vi "PLC_PROXY_MAIN.vi"() -> ()   [LabVIEW 2020]
uses:
  PLC_PROXY/FGV/connection_references/FGV_PROXY_connection_references.ctl
  PLC_PROXY/STATION/station.ctl
  PLC_PROXY/ini/typedef/PROXY_all_config_info.ctl
  PLC_PROXY/ini/typedef/PROXY_main_ini_file.ctl
  PLC_PROXY/queues/typedef/PROXY_queue_refnums.ctl
  PLC_PROXY/queues/typedef/STATION_queue_element.ctl
  PLC_PROXY/STATION/ST_SQL_sequence_state.ctl
  PLC_PROXY/FGV/error_buffer/FGV_PROXY_error_buffer.ctl
  PLC_PROXY/MAIN/PROXY_event_structure_shift_register.ctl
  PLC_PROXY/FGV/DIAGNOSTICS_records_display/FGV_PROXY_DIAGNOSTICS_records_display.ctl
  PLC_PROXY/FGV/DIAGNOSTICS_connection_indicators/FGV_PROXY_connection_indicators.ctl
  PLC_PROXY/FGV/DIAGNOSTICS_message_history_buffer/FGV_PROXY_DIAGNOSTICS_message_history_buffer.ctl
  PLC_PROXY/FGV/SQL_part_ID_buffer/FGV_SQL_part_ID_buffer.ctl
  PLC_PROXY/FGV/SQL_pinion_ID_buffer/FGV_SQL_pinion_ID_buffer.ctl
  PLC_PROXY/FGV/SQL_batch_ID_buffer/FGV_SQL_batch_ID_buffer.ctl
  PLC_PROXY/MAIN/reference_change_listener/PROXY_REF_CHG_sequence_state.ctl
  _misc/NotifyIcon/TypeDefs/NotifyIcon Event Registration Actions.ctl
  _misc/NotifyIcon/TypeDefs/NotifyIcon Events.ctl
  PLC_PROXY/FGV/reference_change_connection/FGV_PROXY_REF_CHG_connection.ctl
  System.Windows.Forms
  _misc/AULocalize/SubVIs/Get Localized Phrase Compact Interface 2D.vi
  _misc/AULocalize/SubVIs/RegisterVI.vi
  _misc/AULocalize/SubVIs/Get Localized Phrase Compact Interface 0D.vi
panel:
  out "app_title":string caption="A603 - PLC Proxy"
  out "SQL_connections_indicator_global":bool=TRUE caption="SQL Connections Status:"
  out "PLC_connections_indicator_global":bool=TRUE caption="PLC Connections Status:"
  in  "STOP":bool
  out "error_indicator_global":bool caption="Application Status:"
  in  "main_tab":enum32{"Diagnostics", "Errors"}(tab)
  in  "DIAGNOSTICS_save_log":bool
  in  "DIAGNOSTICS_all_stations_messages":bool
  in  "DIAGNOSTICS_records":i32(listbox)
  in  "main_error":i32(listbox)
  in  "ERRORS_clear":bool
  out "error_indicator_tab":bool
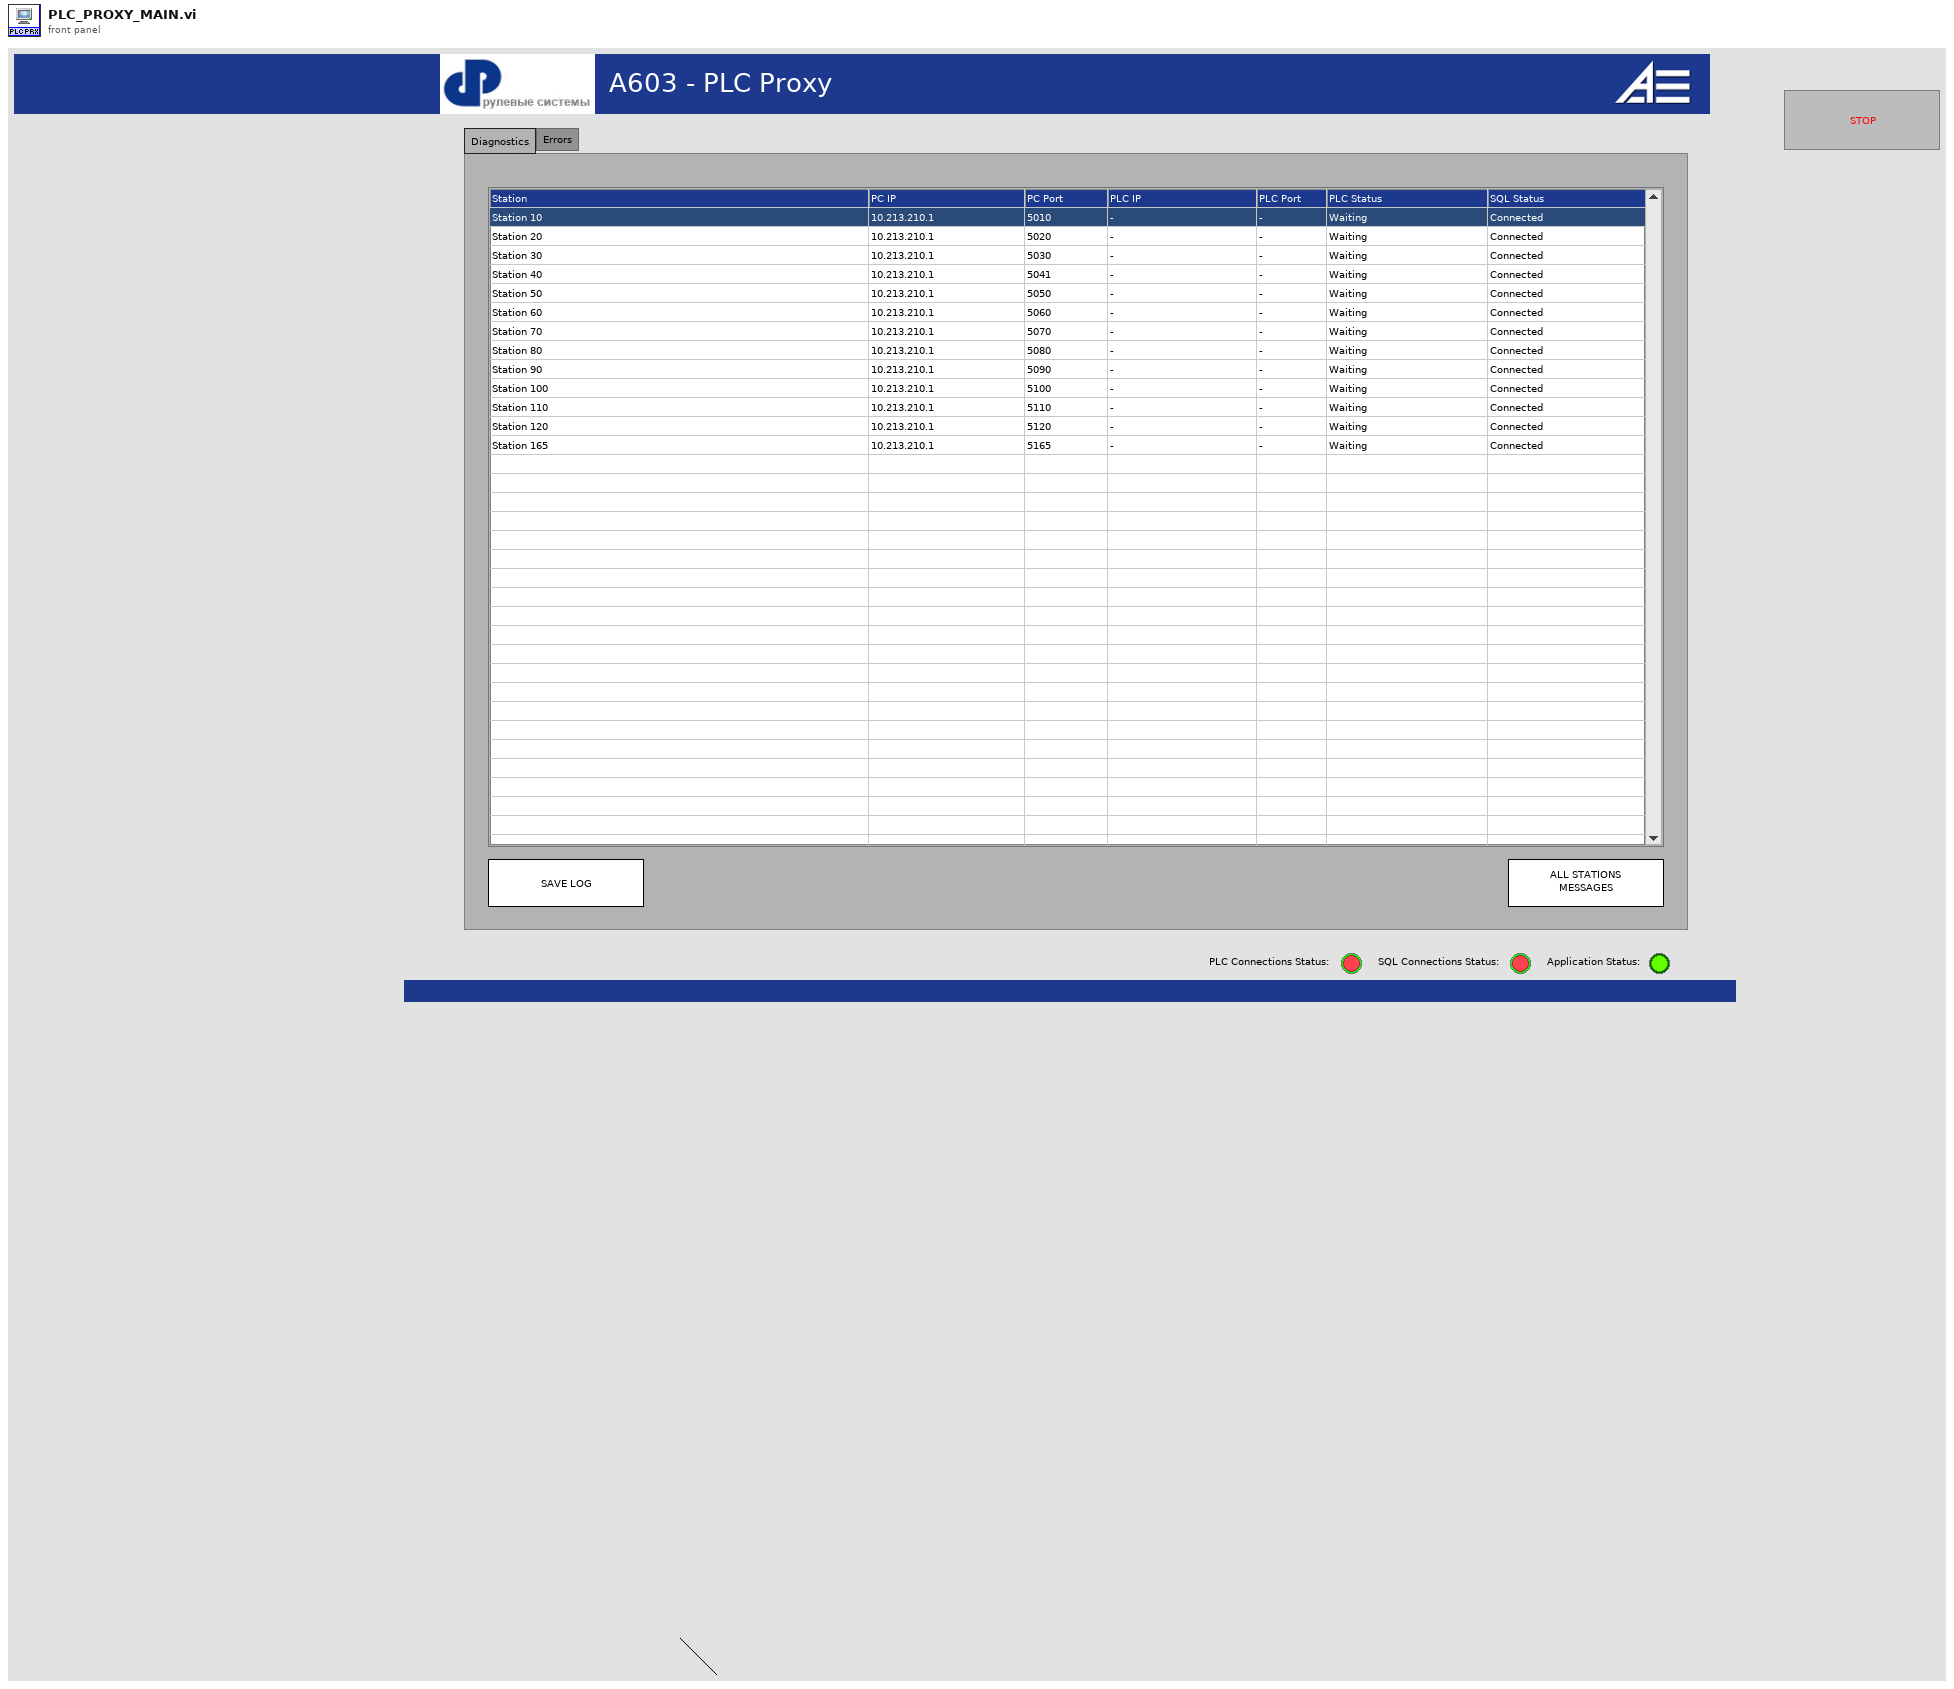
[diagram p1: front panel]
types:
  T1 = typedef "NotifyIcon Events.ctl" = enum16{"BalloonTipClicked", "BalloonTipClosed", "BalloonTipShown", "Click", "Disposed", "DoubleClick", "MouseClick", "MouseDoubleClick", "MouseDown", "MouseMove", "MouseUp", "MenuItemClick", "MenuItemSelect"}
  T2 = typedef "NotifyIcon Event Registration Actions.ctl" = enum16{"Initial Event Registration", "Add to Event Registration", "Destroy Events and Re-register"}
  T3 = typedef "PROXY_REF_CHG_sequence_state.ctl" = enum16{"initialize", "wait_for_connection", "handle_message", "error", "stop"}
  T4 = typedef "FGV_SQL_batch_ID_buffer.ctl" = enum16{"initialize", "get_ID_for_number"}
  T5 = typedef "station.ctl" = enum16{"STATION_10", "STATION_20", "STATION_30", "STATION_40", "STATION_50", "STATION_60", "STATION_70", "STATION_80", "STATION_90", "STATION_100", "STATION_110", "STATION_120", "STATION_165", "MAIN"}
  T6 = typedef "FGV_SQL_pinion_ID_buffer.ctl" = enum16{"initialize", "buffer_pinion_ID", "buffer_pinion_ID_SQL", "get_ID_for_name"}
  T7 = typedef "FGV_SQL_part_ID_buffer.ctl" = enum16{"initialize", "buffer_serial_ID", "get_ID_for_name"}
  T8 = typedef "FGV_PROXY_DIAGNOSTICS_message_history_buffer.ctl" = enum16{"initialize", "add_TCP_PLC_to_PC", "add_TCP_PC_to_PLC", "add_SQL_PC_to_DB", "add_SQL_transaction", "add_SQL_DB_to_PC", "get_station", "get_all", "clear_station", "clear_all", "save_log"}
  T9 = typedef "FGV_PROXY_connection_indicators.ctl" = enum16{"initialize", "SQL_conn_ind_update", "PLC_conn_ind_update"}
  T10 = typedef "FGV_PROXY_DIAGNOSTICS_records_display.ctl" = enum16{"initialize", "set_PLC_IP", "set_PLC_Port", "set_PLC_connection_status", "set_SQL_connection_status", "get_all_info"}
  T11 = typedef "PROXY_event_structure_shift_register.ctl" = cluster{"REF_EDIT_clicked_row":i32, "REF_EDIT_selected_row":i32, "SQL_EDIT_clicked_row":i32, "SQL_EDIT_selected_row":i32, "ARCH_EDIT_selected_row":i32, "ARCH_EDIT_clicked_row":i32, "USER_EDIT_selected_row":i32, "USER_EDIT_clicked_row":i32, "REPORT_GEAR_toggle_all_results":bool}
  T12 = typedef "FGV_PROXY_error_buffer.ctl" = enum16{"initialize", "clear", "display", "get_status"}
  T13 = typedef "PROXY_all_config_info.ctl" = cluster{"main_ini_file":T14, "SQL Password":string, "queue_refnums":T15, "number_of_stations":i32}
  T14 = typedef "PROXY_main_ini_file.ctl" = cluster{"SQL Driver":string, "SQL Server":string, "SQL Database":string, "SQL UID":string, "Reference table":string, "Reference history":string, "Archivisation CFG table":string, "Archivisation CFG history":string, "Archivisation Audit table":string, "User table":string, "User history":string, "default language":string, "REF CHG listener IP":string, "REF CHG listener port":u16, "ST 10 name":string, "ST 10 listener IP":string, "ST 10 listener port":u16, "ST 20 name":string, "ST 20 listener IP":string, "ST 20 listener port":u16, "ST 30 name":string, "ST 30 listener IP":string, "ST 30 listener port":u16, "ST 40 name":string, "ST 40 listener IP":string, "ST 40 listener port":u16, "ST 50 name":string, "ST 50 listener IP":string, "ST 50 listener port":u16, "ST 60 name":string, "ST 60 listener IP":string, "ST 60 listener port":u16, "ST 70 name":string, "ST 70 listener IP":string, "ST 70 listener port":u16, "ST 80 name":string, "ST 80 listener IP":string, "ST 80 listener port":u16, "ST 90 name":string, "ST 90 listener IP":string, "ST 90 listener port":u16, "ST 100 name":string, "ST 100 listener IP":string, "ST 100 listener port":u16, "ST 110 name":string, "ST 110 listener IP":string, "ST 110 listener port":u16, "ST 120 name":string, "ST 120 listener IP":string, "ST 120 listener port":u16, "ST 165 name":string, "ST 165 listener IP":string, "ST 165 listener port":u16}
  T15 = typedef "PROXY_queue_refnums.ctl" = cluster{"ST_10_queue":refnum<queue>, "ST_20_queue":refnum<queue>, "ST_30_queue":refnum<queue>, "ST_40_queue":refnum<queue>, "ST_50_queue":refnum<queue>, "ST_60_queue":refnum<queue>, "ST_70_queue":refnum<queue>, "ST_80_queue":refnum<queue>, "ST_90_queue":refnum<queue>, "ST_100_queue":refnum<queue>, "ST_110_queue":refnum<queue>, "ST_120_queue":refnum<queue>, "ST_165_queue":refnum<queue>}
  T16 = typedef "FGV_PROXY_connection_references.ctl" = enum16{"initialize", "set_listener_ID", "set_connection_ID", "get", "KILL_ALL_CONNECTIONS", "killed?"}
  T17 = typedef "FGV_PROXY_REF_CHG_connection.ctl" = enum16{"initialize", "set_listener_ID", "set_connection_ID", "get", "KILL CONNECTION", "killed?"}
  T18 = enum16{"Standard", "Buffered", "CRLF", "Immediate"}
  T19 = enum32{"Invalid", "Standard", "Closed", "Hidden", "Minimized", "Maximized"}
  T20 = typedef "NotifyIcon Event Data.ctl" = cluster{"NotifyIcon Event":T1, "Data String":string}
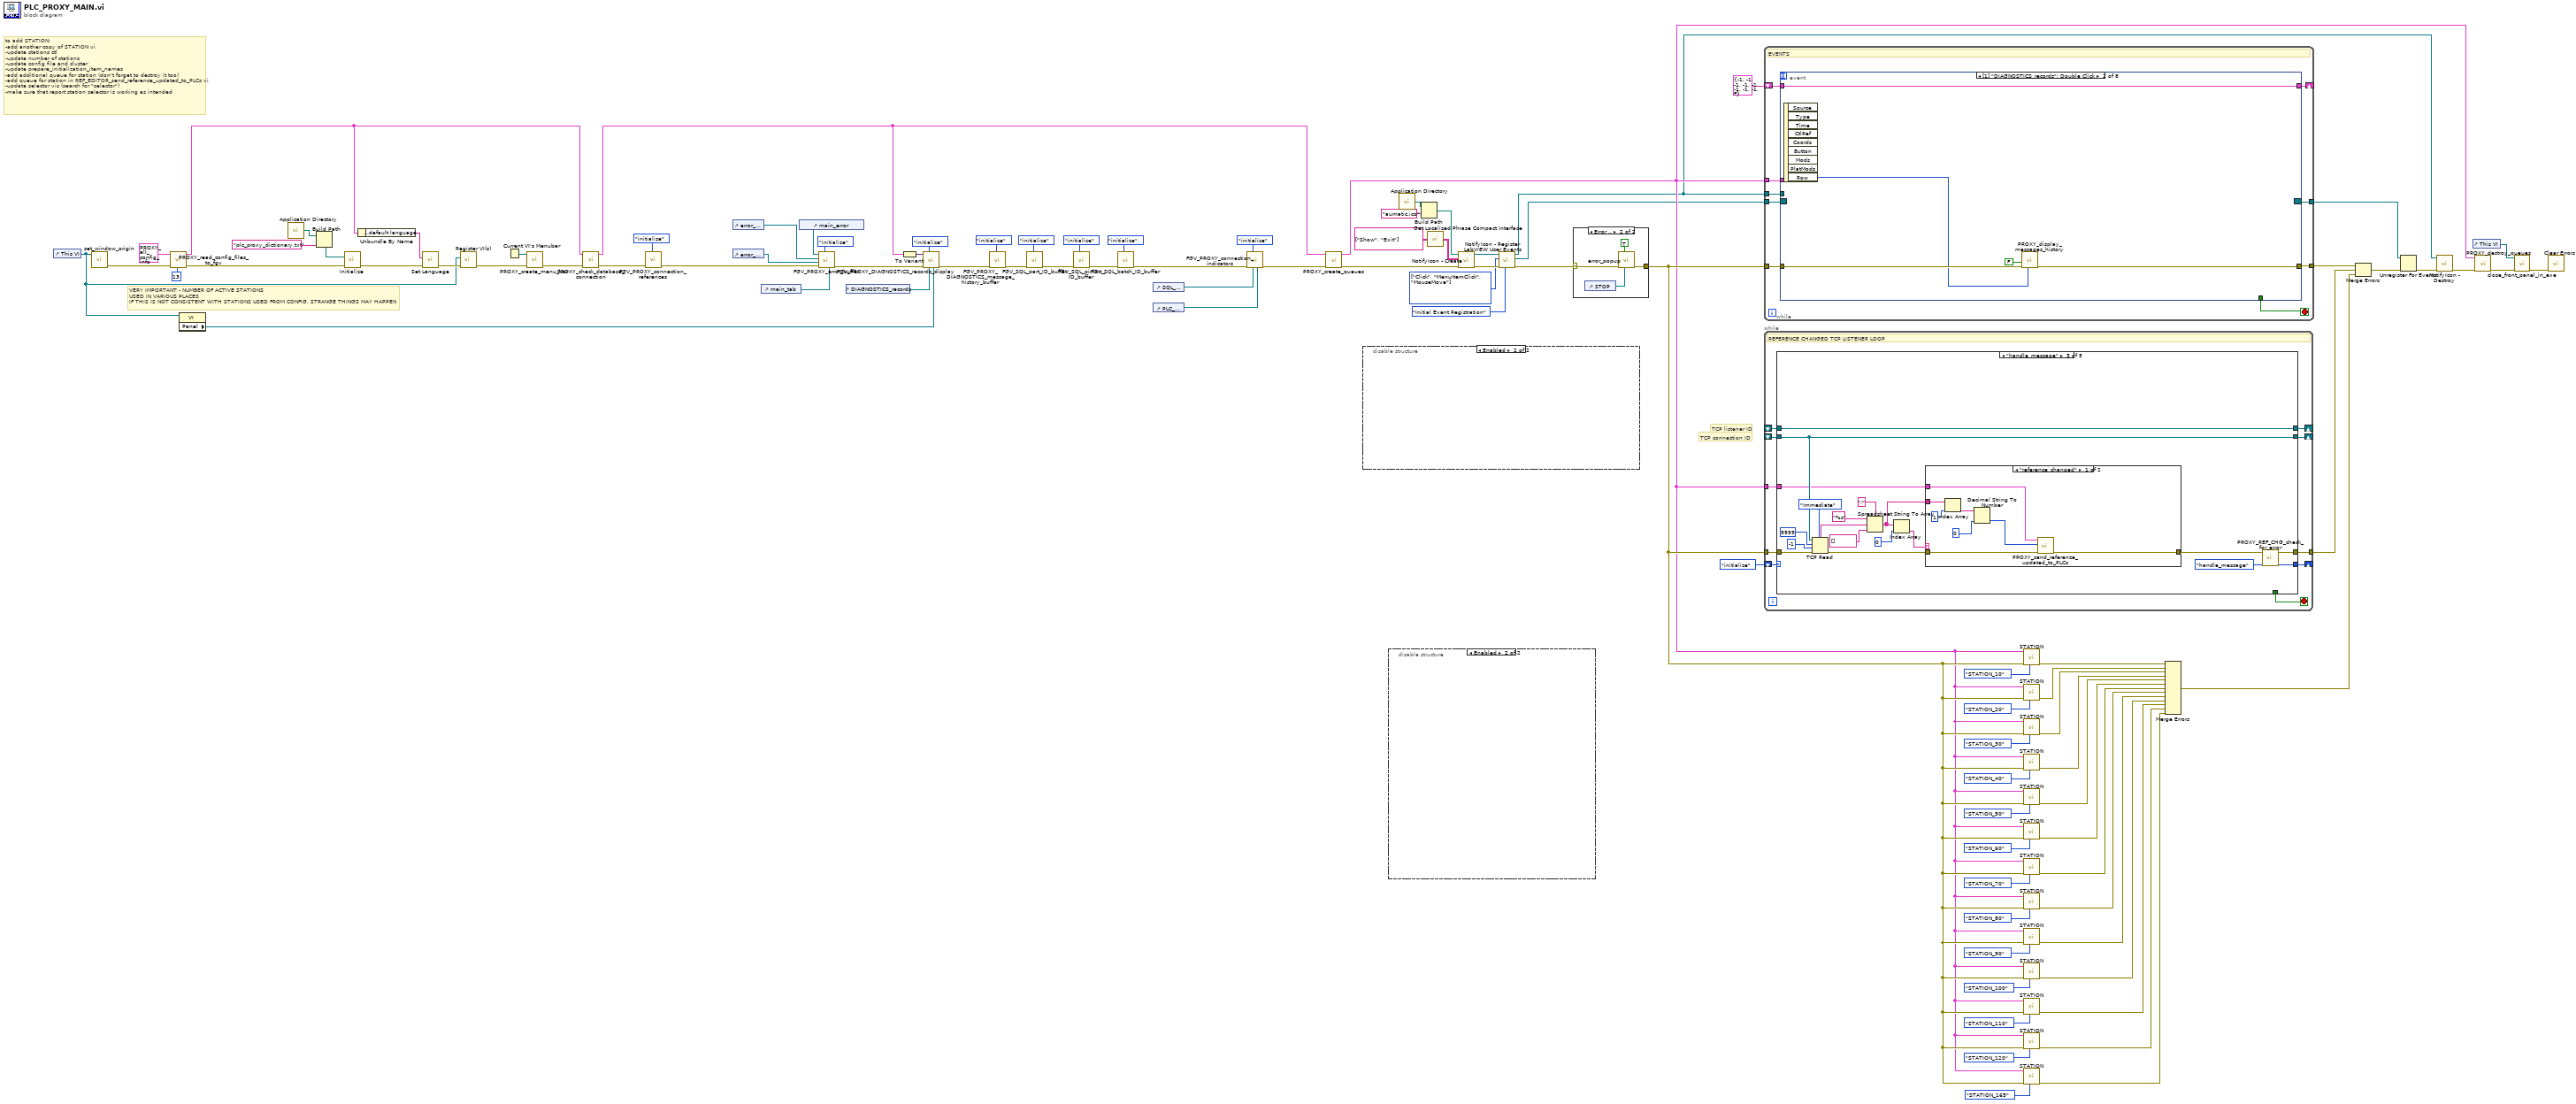
[diagram p0: block diagram]
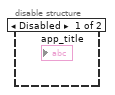
[diagram p2: hidden frame]
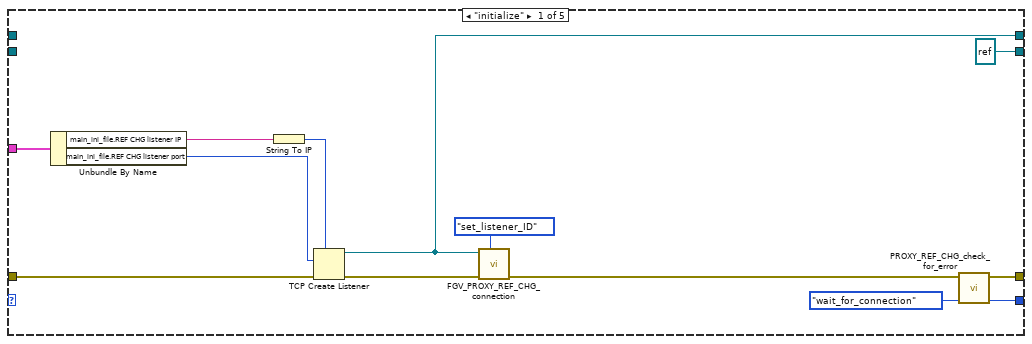
[diagram p3: hidden frame]
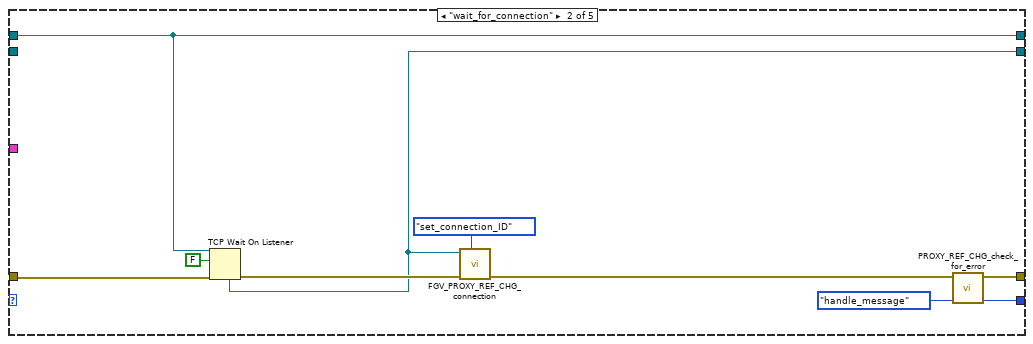
[diagram p4: hidden frame]
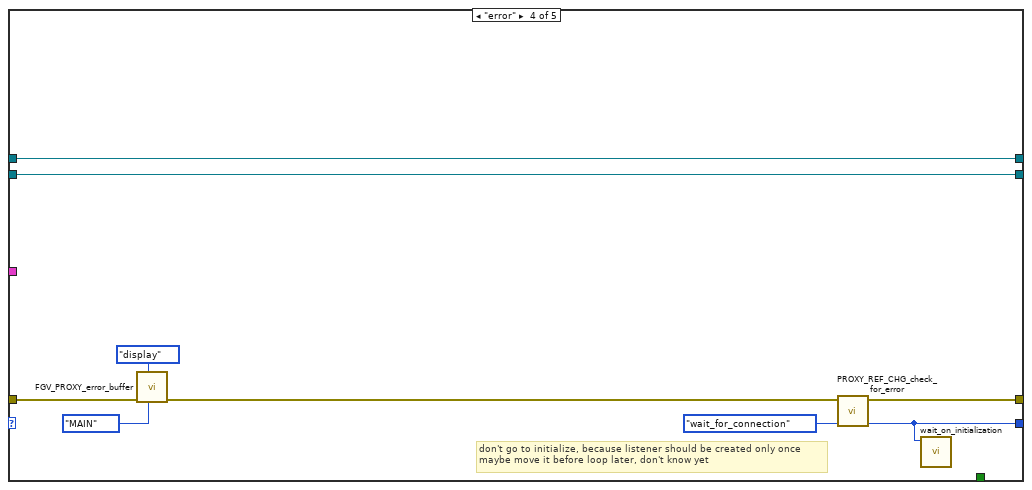
[diagram p6: hidden frame]
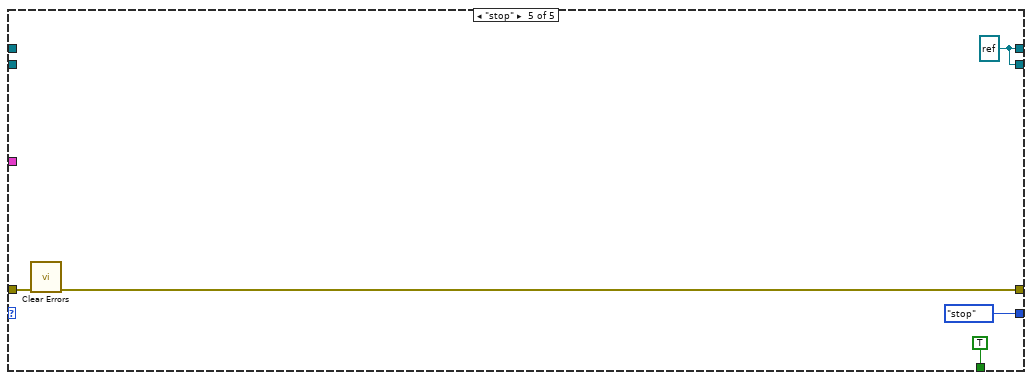
[diagram p7: hidden frame]
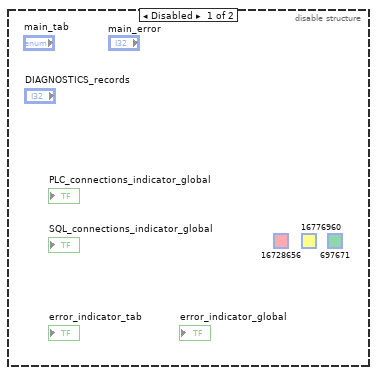
[diagram p9: hidden frame]
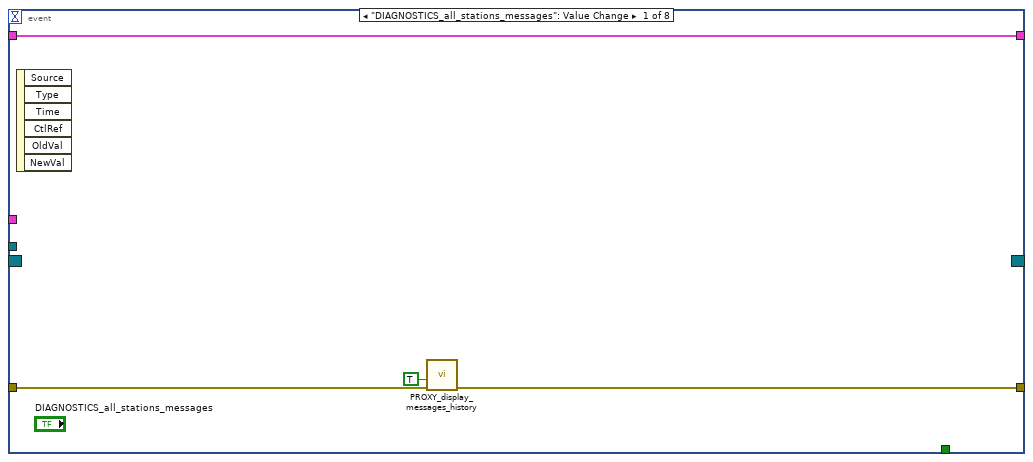
[diagram p10: hidden frame]
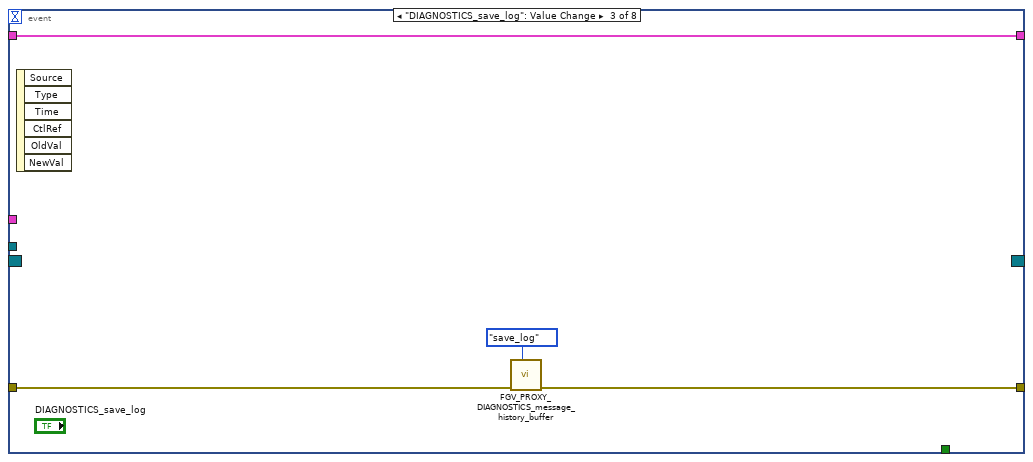
[diagram p11: hidden frame]
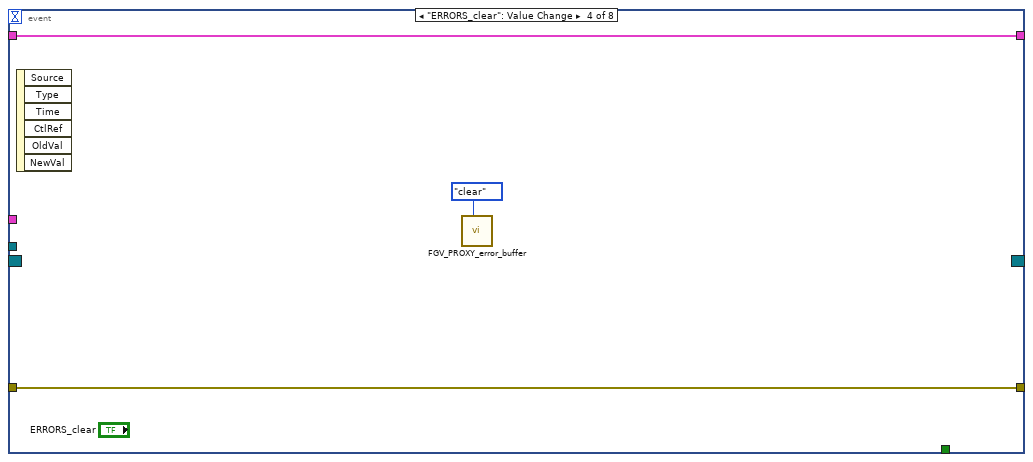
[diagram p12: hidden frame]
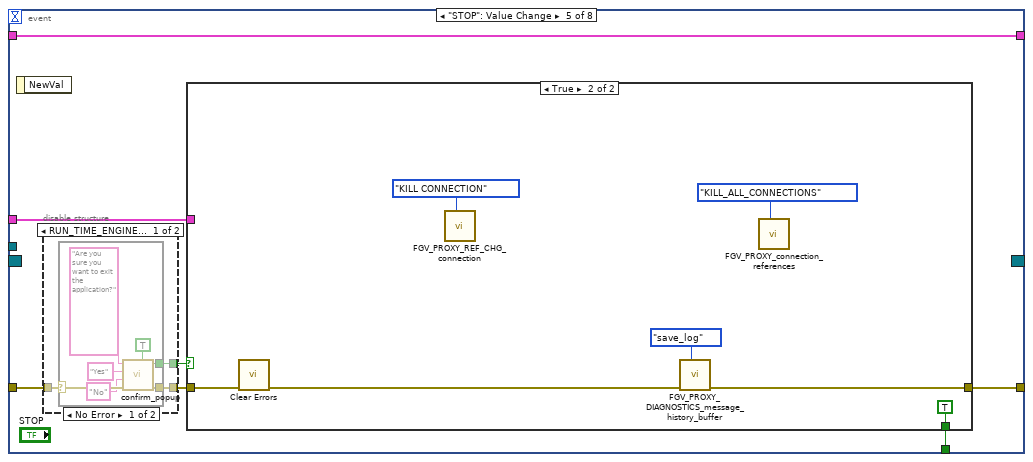
[diagram p13: hidden frame]
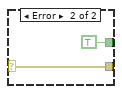
[diagram p14: hidden frame]
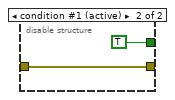
[diagram p15: hidden frame]
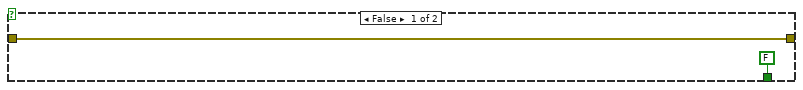
[diagram p16: hidden frame]
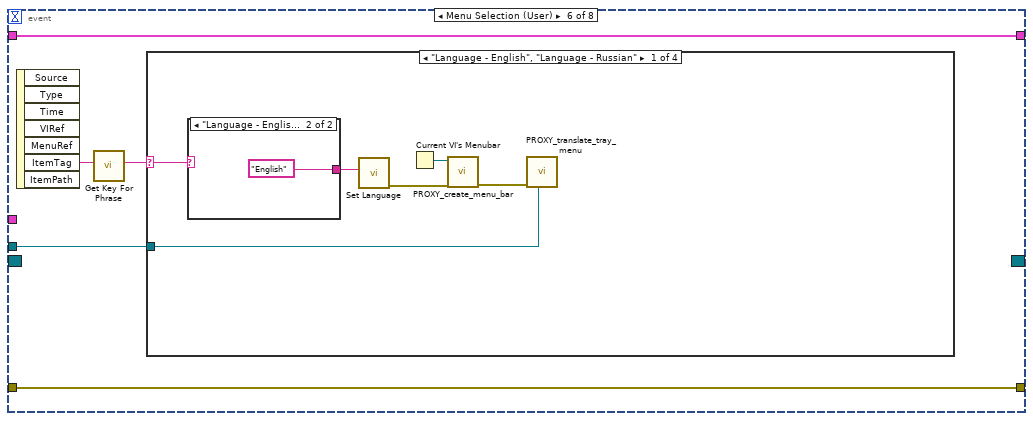
[diagram p17: hidden frame]
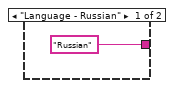
[diagram p18: hidden frame]
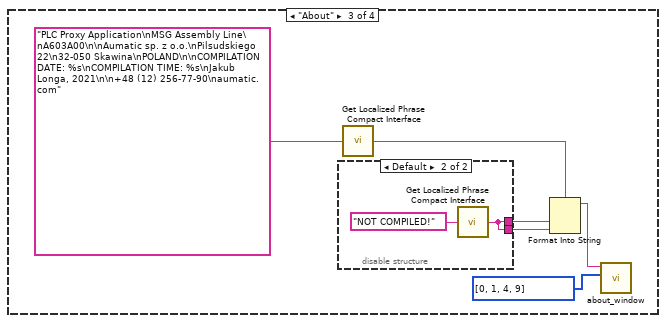
[diagram p20: hidden frame]
diagram:
  w24 = T1[] [enum."Click", enum."MenuItemClick", enum."MouseMove"] items=["BalloonTipClicked", "BalloonTipClosed", "BalloonTipShown", "Click", "Disposed", "DoubleClick", "MouseClick", "MouseDoubleClick", "MouseDown", "MouseMove", "MouseUp", "MenuItemClick", "MenuItemSelect"] ("Events to register")
  # "TCP connection ID"
  # "TCP listener ID"
  # "VERY IMPORTANT - NUMBER OF ACTIVE STATIONS\nUSED IN VARIOUS PLACES\nIF THIS IS NOT CONSISTENT WITH STATIONS USED FROM CONFIG, STRANGE THINGS MAY HAPPEN"
  # "to add STATION:\n-add another copy of STATION vi\n-update stations ctl\n-update number of stations\n-update config file and cluster\n-update prepare_initialization_item_names \n-add additional queue for station (don't forget to destroy it too)\n-add queue for station in REF_EDITOR_send_reference_updated_to_PLCs vi\n-update selector vis (search for \"selector\")\n-make sure that report station selector is working as intended"
  n1 = control-ref of="This VI"() -> (w12:refnum<vi>)
  n2 = call "set_window_origin.vi"("this_vi_reference"=w12) -> ("error_out"=w10:errorcluster)  [unwired: 10 in]
  n3 = call "PROXY_read_config_files_to_fgv.vi"("number_of_stations"=13, "error_in"=w10, "all_config_info_in"=T13 {"main_ini_file"={"SQL Driver"="", "SQL Server"="", "SQL Database"="", "SQL UID"="", "Reference table"="", "Reference history"="", "Archivisation CFG table"="", "Archivisation CFG history"="", "Archivisation Audit table"="", "User table"="", "User history"="", "default language"="", "REF CHG listener IP"="", "REF CHG listener port"=0, "ST 10 name"="", "ST 10 listener IP"="", "ST 10 listener port"=0, "ST 20 name"="", "ST 20 listener IP"="", "ST 20 listener port"=0, "ST 30 name"="", "ST 30 listener IP"="", "ST 30 listener port"=0, "ST 40 name"="", "ST 40 listener IP"="", "ST 40 listener port"=0, "ST 50 name"="", "ST 50 listener IP"="", "ST 50 listener port"=0, "ST 60 name"="", "ST 60 listener IP"="", "ST 60 listener port"=0, "ST 70 name"="", "ST 70 listener IP"="", "ST 70 listener port"=0, "ST 80 name"="", "ST 80 listener IP"="", "ST 80 listener port"=0, "ST 90 name"="", "ST 90 listener IP"="", "ST 90 listener port"=0, "ST 100 name"="", "ST 100 listener IP"="", "ST 100 listener port"=0, "ST 110 name"="", "ST 110 listener IP"="", "ST 110 listener port"=0, "ST 120 name"="", "ST 120 listener IP"="", "ST 120 listener port"=0, "ST 165 name"="", "ST 165 listener IP"="", "ST 165 listener port"=0}, "SQL Password"="", "queue_refnums"={"ST_10_queue"=refnum, "ST_20_queue"=refnum, "ST_30_queue"=refnum, "ST_40_queue"=refnum, "ST_50_queue"=refnum, "ST_60_queue"=refnum, "ST_70_queue"=refnum, "ST_80_queue"=refnum, "ST_90_queue"=refnum, "ST_100_queue"=refnum, "ST_110_queue"=refnum, "ST_120_queue"=refnum, "ST_165_queue"=refnum}, "number_of_stations"=0} ("all_config_info")) -> ("error_out"=w11:errorcluster, "all_config_info_out"=w2:T13)  [unwired: 7 in]
  n4 = property class="VI"(reference=w12) -> ("Panel"=w46:refnum<vi>)  [unwired: 1 in, 2 out]
  n5 = call <vilib>:"Application Directory.vi"() -> ("Application Directory"=w17:path)
  n6 = Build Path(base path=w17, name or relative path="plc_proxy_dictionary.txt") -> (appended path=w15:path)
  n7 = call "Initialize.vi"("Dictionary File Path"=w15, "error in"=w11) -> ("error out"=w14:errorcluster)  [unwired: 8 in, 5 out]
  n8 = Unbundle By Name(w2) -> ("main_ini_file.default language"=w1:string)
  n9 = call "Set Language.vi"("error in"=w14, "Target Language (current lang)"=w1) -> ("error out"=w13:errorcluster)  [unwired: 8 in, 1 out]
  n10 = call-poly "Register VI(s).vi"("error in"=w13, "VI Ref"=w12) -> ("error out"=w8:errorcluster)  [unwired: 8 in, 1 out]
  n11 = Current VI's Menubar() -> (w9:refnum<k9>)
  n12 = call "PROXY_create_menu_bar.vi"("error_in"=w8, "menu_bar_refnum"=w9) -> ("error_out"=w7:errorcluster)  [unwired: 9 in]
  n13 = call "PROXY_check_database_connection.vi"("error_in"=w7, "all_config_info_in"=w2) -> ("error_out"=w6:errorcluster, "all_config_info_out"=w5:T13)  [unwired: 8 in]
  n14 = call "FGV_PROXY_connection_references.vi"("options"=FGV_PROXY_connection_references."initialize", "error_in"=w6) -> ("error_out"=w71:errorcluster)  [unwired: 6 in, 3 out]
  n15 = control-ref of="error_indicator_tab"() -> (w82:refnum<vi>)
  n16 = control-ref of="error_indicator_global"() -> (w81:refnum<vi>)
  n17 = control-ref of="main_tab"() -> (w40:refnum<vi>)
  n18 = control-ref of="main_error"() -> (w90:refnum<vi>)
  n19 = call "FGV_PROXY_error_buffer.vi"("main_tab"=w40, "option"=FGV_PROXY_error_buffer."initialize", "error_in"=w71, "error_indicator_global"=w81, "error_indicator_tab"=w82, "error_display_ref"=w90) -> ("error_out"=w79:errorcluster)  [unwired: 4 in, 1 out]
  n20 = control-ref of="DIAGNOSTICS_records"() -> (w78:refnum<vi>)
  n21 = To Variant(anything=w5) -> (Variant=w77:variant)
  n22 = call "FGV_PROXY_DIAGNOSTICS_records_display.vi"("front_panel_reference"=w46, "SQL_listbox_reference"=w78, "options"=FGV_PROXY_DIAGNOSTICS_records_display."initialize", "error_in"=w79, "input"=w77) -> ("error_out"=w39:errorcluster)  [unwired: 5 in, 1 out]
  n23 = call "FGV_PROXY_DIAGNOSTICS_message_history_buffer.vi"("options"=FGV_PROXY_DIAGNOSTICS_message_history_buffer."initialize", "error_in"=w39) -> ("error_out"=w69:errorcluster)  [unwired: 8 in, 1 out]
  n24 = call "FGV_SQL_part_ID_buffer.vi"("options"=FGV_SQL_part_ID_buffer."initialize", "error_in"=w69) -> ("error_out"=w47:errorcluster)  [unwired: 7 in, 2 out]
  n25 = call "FGV_SQL_pinion_ID_buffer.vi"("options"=FGV_SQL_pinion_ID_buffer."initialize", "error_in"=w47) -> ("error_out"=w43:errorcluster)  [unwired: 7 in, 2 out]
  n26 = call "FGV_SQL_batch_ID_buffer.vi"("options"=FGV_SQL_batch_ID_buffer."initialize", "error_in"=w43) -> ("error_out"=w42:errorcluster)  [unwired: 7 in, 2 out]
  n27 = control-ref of="SQL_connections_indicator_global"() -> (w74:refnum<vi>)
  n28 = control-ref of="PLC_connections_indicator_global"() -> (w73:refnum<vi>)
  n29 = call "FGV_PROXY_connection_indicators.vi"("PLC_connections_indicator_global"=w73, "SQL_connections_indicator_global"=w74, "options"=FGV_PROXY_connection_indicators."initialize", "error_in"=w42) -> ("error_out"=w76:errorcluster)  [unwired: 7 in]
  n30 = call "PROXY_create_queues.vi"("error_in"=w76, "all_config_info_in"=w5) -> ("error_out"=w31:errorcluster, "all_config_info_out"=w35:T13)  [unwired: 8 in]
  n31 = disable-structure shown="Enabled" {
    frame Disabled {
    }
    frame Enabled {
    }
  }
  n32 = disable-structure shown="Enabled" {
    frame Disabled {
      (unwired) u32 16728656
      (unwired) u32 16776960
      (unwired) u32 697671
    }
    frame Enabled {
    }
  }
  n33 = call <vilib>:"Application Directory.vi"() -> ("Application Directory"=w33:path)
  n34 = Build Path(base path=w33, name or relative path="aumatic.ico" ("icon_name")) -> (appended path=w27:path)
  n35 = call-poly "Get Localized Phrase Compact Interface.vi"("Key"=string[][] [["Show"], ["Exit"]] ("Context Menu (optional)")) -> ("Translated Phrase"=w4:string[][])
  n36 = call "NotifyIcon - Create.vi"("error in"=w31, "Context Menu (optional)"=w4, "Icon File Path"=w27) -> ("error out"=w30:errorcluster, "NotifyIcon reference"=w26:refnum<k24>)  [unwired: 7 in]
  n37 = call "NotifyIcon - Register LabVIEW User Events.vi"("Action"=NotifyIcon_Event_Registration_Actions."Initial Event Registration", "error in"=w30, "Events to register"=w24, "NotifyIcon reference in"=w26) -> ("error out"=w29:errorcluster, "Event Registration Refnum"=w23:refnum<event-registration>, "NotifyIcon reference out"=w3:refnum<k24>)  [unwired: 5 in]
  n38 = case shown="Error .." w29 {
    selector: w29 -> [w96 w99]
    tunnel: [w96 w100] -> w37
    frame No Error {
    }
    frame Error {
      n39 = control-ref of="STOP"() -> (w98:refnum<vi>)
      n40 = call "error_popup.vi"("STOP_button_reference"=w98, "EXIT App If Error? (F)"=TRUE, "error_in"=w99) -> ("error_out"=w100:errorcluster)  [unwired: 8 in]
    }
  }
  n41 = while {
    shift-right: [w109] -> _
    shift-left: _ -> [w108]
    shift-right: [w107] -> _
    shift-left: _ -> [w106]
    tunnel: w37 -> [w105]
    tunnel: [w104] -> w36
    tunnel: w35 -> [w103]
    shift-right: [w101] -> _
    shift-left: PROXY_REF_CHG_sequence_state."initialize" ("ST_TCP_sequence_state") -> [w102]
    stop <- w110 stop-if-true
    # "REFERENCE CHANGED TCP LISTENER LOOP"
    n42 = case shown="\"handle_message\"" w102 {
      tunnel: [_ _ _ _ TRUE] -> w110
      tunnel: [w122 w132 w149 w170 w171] -> w104
      tunnel: [w111 w129 w152 w166 w173] -> w109
      tunnel: w108 -> [_ w129 w152 w166 _]
      tunnel: [w121 w130 w148 w167 PROXY_REF_CHG_sequence_state."stop" ("PLC_TCP_loop_state_in")] -> w101
      tunnel: [refnum<k5> refnum ("connection ID") w125 w142 w165 w173] -> w107
      tunnel: w106 -> [_ _ w142 w165 _]
      tunnel: w105 -> [w118 w128 w145 w164 w172]
      tunnel: w103 -> [w117 _ w141 _ _]
      frame "initialize" {
        n43 = Unbundle By Name(w117) -> ("main_ini_file.REF CHG listener IP"=w116:string, "main_ini_file.REF CHG listener port"=w115:u16)
        n44 = String To IP(1:w116) -> (0:w123:u32)
        n45 = TCP Create Listener(7:w123, 8:w118, 10:w115) -> (0:w114:errorcluster, 3:w111:refnum<k5>)  [unwired: 2 in, 1 out]
        n46 = call "FGV_PROXY_REF_CHG_connection.vi"("options"=FGV_PROXY_REF_CHG_connection."set_listener_ID", "error_in"=w114, "reference_in"=w111) -> ("error_out"=w113:errorcluster)  [unwired: 5 in, 3 out]
        n47 = call "PROXY_REF_CHG_check_for_error.vi"("PROXY_REF_CHG_sequence_state_in"=PROXY_REF_CHG_sequence_state."wait_for_connection" ("PLC_TCP_loop_state_in"), "error_in"=w113) -> ("PROXY_REF_CHG_sequence_state_out"=w121:T3, "error_out"=w122:errorcluster)  [unwired: 8 in]
      }
      frame "wait_for_connection" {
        n48 = TCP Wait On Listener(8:w128, 10:FALSE ("resolve remote address (T)"), 11:w129) -> (0:w127:errorcluster, 4:w125:refnum<k5>)  [unwired: 1 in, 3 out]
        n49 = call "FGV_PROXY_REF_CHG_connection.vi"("options"=FGV_PROXY_REF_CHG_connection."set_connection_ID", "error_in"=w127, "reference_in"=w125) -> ("error_out"=w124:errorcluster)  [unwired: 5 in, 3 out]
        n50 = call "PROXY_REF_CHG_check_for_error.vi"("PROXY_REF_CHG_sequence_state_in"=PROXY_REF_CHG_sequence_state."handle_message" ("PLC_TCP_1_loop_states"), "error_in"=w124) -> ("PROXY_REF_CHG_sequence_state_out"=w130:T3, "error_out"=w132:errorcluster)  [unwired: 8 in]
      }
      frame "handle_message" {
        n51 = TCP Read(connection ID=w142, bytes to read=9999, error in (no error)=w145, 7:T18."Immediate" ("mode (standard)"), 9:-1 ("timeout ms (25000)")) -> (data out=w138:string, error out=w144:errorcluster)  [unwired: 1 out]
        n52 = Spreadsheet String To Array(delimiter (Tab)=";", format string="%s", spreadsheet string=w138, array type (2D Dbl)=string[] []) -> (array=w134:string[])
        n53 = Index Array(array=w134, index=0 ("timeout ms (25000)")) -> (element=w135:string)
        n54 = case shown="\"reference_changed\"" w135 {
          tunnel: w144 -> [w160 w161]
          tunnel: [w159 w161] -> w143
          tunnel: w141 -> [w158 _]
          tunnel: w134 -> [w156 _]
          frame "reference_changed" {
            n55 = Index Array(array=w156, index=1 ("timeout ms (25000)")) -> (element=w155:string)
            n56 = Decimal String To Number(string=w155, default (0L)=0 ("timeout ms (25000)")) -> (number=w153:i32)  [unwired: 1 in, 1 out]
            n57 = call "PROXY_send_reference_updated_to_PLCs.vi"("error_in"=w160, "num_station"=w153, "all_config_info_out"=w158) -> ("error_out"=w159:errorcluster)  [unwired: 8 in]
          }
          frame Default {
          }
        }
        n58 = call "PROXY_REF_CHG_check_for_error.vi"("PROXY_REF_CHG_sequence_state_in"=PROXY_REF_CHG_sequence_state."handle_message" ("PLC_TCP_loop_state_in"), "error_in"=w143) -> ("PROXY_REF_CHG_sequence_state_out"=w148:T3, "error_out"=w149:errorcluster)  [unwired: 8 in]
      }
      frame "error" {
        # "don't go to initialize, because listener should be created only once\nmaybe move it before loop later, don't know yet"
        n59 = call "FGV_PROXY_error_buffer.vi"("station"=station."MAIN", "option"=FGV_PROXY_error_buffer."display", "error_in"=w164) -> ("error_out"=w163:errorcluster)  [unwired: 7 in, 1 out]
        n60 = call "PROXY_REF_CHG_check_for_error.vi"("PROXY_REF_CHG_sequence_state_in"=PROXY_REF_CHG_sequence_state."wait_for_connection" ("PLC_TCP_loop_state_in"), "error_in"=w163) -> ("PROXY_REF_CHG_sequence_state_out"=w167:T3, "error_out"=w170:errorcluster)  [unwired: 8 in]
        n61 = call "wait_on_initialization.vi"("state"=w167) -> ()  [unwired: 11 in]
      }
      frame "stop" {
        w173 = refnum<k5> refnum ("connection ID")
        n62 = call <vilib>:"Clear Errors.vi"("error in (no error)"=w172) -> ("error out"=w171:errorcluster)  [unwired: 5 in, 1 out]
      }
    }
  }
  n63 = while {
    tunnel: w37 -> [w183]
    tunnel: [w184] -> w84
    tunnel: w35 -> [w181]
    shift-right: [w180] -> _
    shift-left: T11 {"REF_EDIT_clicked_row"=-1, "REF_EDIT_selected_row"=-1, "SQL_EDIT_clicked_row"=-1, "SQL_EDIT_selected_row"=-1, "ARCH_EDIT_selected_row"=-1, "ARCH_EDIT_clicked_row"=-1, "USER_EDIT_selected_row"=-1, "USER_EDIT_clicked_row"=-1, "REPORT_GEAR_toggle_all_results"=FALSE} -> [w179]
    tunnel: w23 -> [w178]
    tunnel: [w177] -> w19
    tunnel: w3 -> [w176]
    stop <- w182 stop-if-true
    # "EVENTS"
    n64 = event shown="[1] \"DIAGNOSTICS_records\": Double Click" {
      selector: w178 -> [_ _ _ _ _ _ _ _]
      dyn-events: [_ _ _ _ _ _ _ _] -> w177
      timeout: _ -> [_ _ _ _ _ _ _ _]
      tunnel: [_ _ _ _ w201 _ _ _] -> w182
      tunnel: w183 -> [w187 w192 w195 w200 w204 w235 w263 w295]
      tunnel: [w186 w191 w194 w200 w205 w235 w257 w288] -> w184
      tunnel: w181 -> [_ _ _ _ w207 _ _ _]
      tunnel: [w188 w193 w197 w198 w206 w234 w264 w297] -> w180
      tunnel: w179 -> [w188 w193 w197 w198 w206 w234 w264 w297]
      tunnel: w176 -> [_ _ _ _ _ w231 w256 w291]
      event "DIAGNOSTICS_all_stations_messages": Value Change {
        n65 = event-data() -> ()  [unwired: 1 in, 6 out]
        n66 = call "PROXY_display_messages_history.vi"("error_in"=w187, "All Stations?"=TRUE) -> ("error_out"=w186:errorcluster)  [unwired: 9 in]
      }
      event "DIAGNOSTICS_records": Double Click {
        n67 = event-data() -> ("Row"=w189:i32)  [unwired: 1 in, 8 out]
        n68 = call "PROXY_display_messages_history.vi"("station_in"=w189, "error_in"=w192, "All Stations?"=FALSE) -> ("error_out"=w191:errorcluster)  [unwired: 8 in]
      }
      event "DIAGNOSTICS_save_log": Value Change {
        n69 = event-data() -> ()  [unwired: 1 in, 6 out]
        n70 = call "FGV_PROXY_DIAGNOSTICS_message_history_buffer.vi"("options"=FGV_PROXY_DIAGNOSTICS_message_history_buffer."save_log", "error_in"=w195) -> ("error_out"=w194:errorcluster)  [unwired: 8 in, 1 out]
      }
      event "ERRORS_clear": Value Change {
        n71 = event-data() -> ()  [unwired: 1 in, 6 out]
        n72 = call "FGV_PROXY_error_buffer.vi"("option"=FGV_PROXY_error_buffer."clear") -> ()  [unwired: 9 in, 2 out]
      }
      event "STOP": Value Change {
        n73 = event-data() -> ()  [unwired: 1 in, 1 out]
        n74 = disable-structure shown="RUN_TIME_ENGINE==True" {
          disable-tunnel: [w210 TRUE ("Result")] -> w202
          disable-tunnel: w204 -> [w209 w221]
          disable-tunnel: [w208 w221] -> w203
          frame condition #0 {
            n75 = case shown="No Error" w209 {
              selector: w209 -> [w215 w219]
              tunnel: [w216 TRUE ("Result")] -> w210
              tunnel: [w214 w219] -> w208
              frame No Error {
                n76 = call "confirm_popup.vi"("Warning(T)/Inf(F)"=TRUE, "error_in"=w215, "False Label"="No", "True Label"="Yes", "Message"="Are you sure you want to exit the application?") -> ("error_out"=w214:errorcluster, "Result"=w216:bool)  [unwired: 5 in]
              }
              frame Error {
              }
            }
          }
          frame condition #1 (active) {
          }
        }
        n77 = case shown="True" w202 {
          tunnel: w207 -> [_ _]
          tunnel: w203 -> [w223 w230]
          tunnel: [w223 w228] -> w205
          tunnel: [FALSE TRUE] -> w201
          frame False {
          }
          frame True {
            n78 = call <vilib>:"Clear Errors.vi"("error in (no error)"=w230) -> ("error out"=w225:errorcluster)  [unwired: 5 in, 1 out]
            n79 = call "FGV_PROXY_REF_CHG_connection.vi"("options"=FGV_PROXY_REF_CHG_connection."KILL CONNECTION") -> ()  [unwired: 7 in, 4 out]
            n80 = call "FGV_PROXY_DIAGNOSTICS_message_history_buffer.vi"("options"=FGV_PROXY_DIAGNOSTICS_message_history_buffer."save_log", "error_in"=w225) -> ("error_out"=w228:errorcluster)  [unwired: 8 in, 1 out]
            n81 = call "FGV_PROXY_connection_references.vi"("options"=FGV_PROXY_connection_references."KILL_ALL_CONNECTIONS") -> ()  [unwired: 7 in, 4 out]
          }
        }
      }
      event Menu Selection (User) {
        n82 = event-data() -> ("ItemTag"=w233:string)  [unwired: 1 in, 6 out]
        n83 = call "Get Key For Phrase.vi"("Phrase"=w233) -> ("Key"=w232:string)  [unwired: 9 in, 1 out]
        n84 = case shown="\"Language - English\", \"Language - Russian\"" w232 {
          selector: w232 -> [w240 _ _ _]
          tunnel: w231 -> [w236 _ _ _]
          frame "Language - English", "Language - Russian" {
            n85 = case shown="\"Language - English\", Default" w240 {
              tunnel: ["Russian" ("Target Language (current lang)") "English" ("Target Language (current lang)")] -> w241
              frame "Language - Russian" {
              }
              frame "Language - English", Default {
              }
            }
            n86 = call "Set Language.vi"("Target Language (current lang)"=w241) -> ("error out"=w238:errorcluster)  [unwired: 9 in, 1 out]
            n87 = Current VI's Menubar() -> (w239:refnum<k9>)
            n88 = call "PROXY_create_menu_bar.vi"("error_in"=w238, "menu_bar_refnum"=w239) -> ("error_out"=w237:errorcluster)  [unwired: 9 in]
            n89 = call "PROXY_translate_tray_menu.vi"("NotifyIcon reference in"=w236, "error_in"=w237) -> ()  [unwired: 9 in, 1 out]
          }
          frame Default {
          }
          frame "About" {
            n90 = disable-structure shown="Default" {
              disable-tunnel: [w250 w253] -> w246
              disable-tunnel: [w251 w253] -> w245
              frame condition #0 {
                n91 = vi-ref "get_exe_compilation_date.vi"() -> (w252:refnum<vi>)
                n92 = call-by-ref "?"(reference=w252) -> ("compilation_time"=w250:string, "compilation_date"=w251:string)  [unwired: 10 in, 3 out]
              }
              frame condition #1 (active) {
                n93 = call-poly "Get Localized Phrase Compact Interface.vi"("Key"="NOT COMPILED!" ("compilation_date")) -> ("Translated Phrase"=w253:string)
              }
            }
            n94 = call-poly "Get Localized Phrase Compact Interface.vi"("Key"="PLC Proxy Application\nMSG Assembly Line\nA603A00\n\nAumatic sp. z o.o.\nPilsudskiego 22\n32-050 Skawina\nPOLAND\n\nCOMPILATION DATE: %s\nCOMPILATION TIME: %s\nJakub Longa, 2021\n\n+48 (12) 256-77-90\naumatic.com" ("about_string")) -> ("Translated Phrase"=w244:string)
            n95 = Format Into String(format string=w244, w245, w246) -> (resulting string=w249:string)  [unwired: 2 in, 1 out]
            n96 = call "about_window.vi"("lines_to_bold"=i32[] [0, 1, 4, 9], "about_string"=w249) -> ()  [unwired: 9 in, 1 out]
          }
          frame "Exit" {
            n97 = property on="STOP" class="Bool (strict)"("Val(Sgnl)"=TRUE ("Value (Signaling)")) -> ()  [unwired: 2 in, 2 out]
          }
        }
      }
      event User Event {
        n98 = event-data() -> ("Event Data"=w262:variant)  [unwired: 1 in]
        n99 = call "NotifyIcon - Interpret Event Data.vi"("error in"=w263, "NotifyIcon Event Data"=w262) -> ("error out"=w260:errorcluster, "NotifyIcon Event Data"=w261:T20)  [unwired: 8 in]
        n100 = Unbundle By Name(w261) -> ("NotifyIcon Event"=w259:T1, "Data String"=w258:string)
        n101 = case shown="\"MenuItemClick\"" w259 {
          tunnel: w260 -> [w266 w272 w284 w285]
          tunnel: w258 -> [_ w270 _ _]
          tunnel: [w265 w271 w282 w285] -> w257
          tunnel: w256 -> [_ _ w283 _]
          frame "Click" {
            n102 = invoke class="VI" method="FP.Open"(error in=w266, "Activate"=TRUE ("Activate?"), "State"=T19."Standard") -> (error out=w265:errorcluster)  [unwired: 2 in, 4 out]
          }
          frame "MenuItemClick" {
            n103 = call "Get Key For Phrase.vi"("Phrase"=w270) -> ("Key"=w269:string)  [unwired: 9 in, 1 out]
            n104 = case shown="\"Exit\"" w269 {
              tunnel: w272 -> [w273 w275 w277]
              tunnel: [w273 w275 w276] -> w271
              frame "Exit" {
                n105 = property on="STOP" class="Bool (strict)"("Val(Sgnl)"=TRUE ("Value (Signaling)")) -> ()  [unwired: 2 in, 2 out]
              }
              frame Default {
              }
              frame "Show" {
                n106 = invoke class="VI" method="FP.Open"(error in=w277, "Activate"=TRUE ("Activate?"), "State"=T19."Standard") -> (error out=w276:errorcluster)  [unwired: 2 in, 4 out]
              }
            }
          }
          frame "MouseMove" {
            n107 = call-poly "Get Localized Phrase Compact Interface.vi"("Key"="PLC Proxy" ("Text")) -> ("Translated Phrase"=w280:string)
            n108 = property class="NotifyIcon"(reference=w283, error in=w284, "Text"=w280) -> (error out=w282:errorcluster)  [unwired: 1 out]
          }
          frame Default {
          }
        }
      }
      event Panel Close? {
        w293 = 1 items=["None", "Info", "Warning", "Error"] ("Icon (None)")
        n109 = event-data() -> ()  [unwired: 1 in, 4 out]
        n110 = property class="VI"(error in=w295, "FP.State"=T19."Hidden" ("Front Panel Window:State")) -> (error out=w294:errorcluster)  [unwired: 1 in, 1 out]
        n111 = call-poly "Get Localized Phrase Compact Interface.vi"("Key"="PLC Proxy" ("Title")) -> ("Translated Phrase"=w287:string)
        n112 = call-poly "Get Localized Phrase Compact Interface.vi"("Key"="Minimized to tray" ("Text")) -> ("Translated Phrase"=w286:string)
        n113 = call "NotifyIcon - Show BalloonTip.vi"("display time (ms)"=5000, "Icon (None)"=w293, "error in"=w294, "Text"=w286, "Title"=w287, "NotifyIcon reference in"=w291) -> ("error out"=w288:errorcluster)  [unwired: 4 in, 1 out]
        n114 = event-data("Discard?"=TRUE) -> ()  [unwired: 1 in, 1 out]
      }
    }
  }
  n115 = call "STATION.vi"("station"=station."STATION_10", "error_in"=w37, "all_config_info"=w35) -> ("error_out"=w87:errorcluster)  [unwired: 8 in]
  n116 = call "STATION.vi"("station"=station."STATION_20" ("stations"), "error_in"=w37, "all_config_info"=w35) -> ("error_out"=w86:errorcluster)  [unwired: 8 in]
  n117 = call "STATION.vi"("station"=station."STATION_30" ("stations"), "error_in"=w37, "all_config_info"=w35) -> ("error_out"=w85:errorcluster)  [unwired: 8 in]
  n118 = call "STATION.vi"("station"=station."STATION_40" ("stations"), "error_in"=w37, "all_config_info"=w35) -> ("error_out"=w58:errorcluster)  [unwired: 8 in]
  n119 = call "STATION.vi"("station"=station."STATION_50" ("stations"), "error_in"=w37, "all_config_info"=w35) -> ("error_out"=w59:errorcluster)  [unwired: 8 in]
  n120 = call "STATION.vi"("station"=station."STATION_60" ("stations"), "error_in"=w37, "all_config_info"=w35) -> ("error_out"=w18:errorcluster)  [unwired: 8 in]
  n121 = call "STATION.vi"("station"=station."STATION_70" ("stations"), "error_in"=w37, "all_config_info"=w35) -> ("error_out"=w60:errorcluster)  [unwired: 8 in]
  n122 = call "STATION.vi"("station"=station."STATION_80" ("stations"), "error_in"=w37, "all_config_info"=w35) -> ("error_out"=w61:errorcluster)  [unwired: 8 in]
  n123 = call "STATION.vi"("station"=station."STATION_90" ("stations"), "error_in"=w37, "all_config_info"=w35) -> ("error_out"=w62:errorcluster)  [unwired: 8 in]
  n124 = call "STATION.vi"("station"=station."STATION_100" ("stations"), "error_in"=w37, "all_config_info"=w35) -> ("error_out"=w63:errorcluster)  [unwired: 8 in]
  n125 = call "STATION.vi"("station"=station."STATION_110" ("stations"), "error_in"=w37, "all_config_info"=w35) -> ("error_out"=w64:errorcluster)  [unwired: 8 in]
  n126 = call "STATION.vi"("station"=station."STATION_120" ("stations"), "error_in"=w37, "all_config_info"=w35) -> ("error_out"=w65:errorcluster)  [unwired: 8 in]
  n127 = call "STATION.vi"("station"=station."STATION_165", "error_in"=w37, "all_config_info"=w35) -> ("error_out"=w45:errorcluster)  [unwired: 8 in]
  n128 = Merge Errors(w87, w86, w85, w58, w59, w18, w60, w61, w62, w63, w64, w65, w45) -> (w38:errorcluster)
  n129 = Merge Errors(w84, w36, w38) -> (w21:errorcluster)
  n130 = Unregister For Events(event registration refnum=w19, error in=w21) -> (error out=w20:errorcluster)
  n131 = call "NotifyIcon - Destroy.vi"("error in"=w20, "NotifyIcon reference"=w3) -> ("error out"=w22:errorcluster)  [unwired: 9 in]
  n132 = control-ref of="This VI"() -> (w92:refnum<vi>)
  n133 = call "PROXY_destroy_queues.vi"("error_in"=w22, "all_config_info"=w35) -> ("error_out"=w93:errorcluster)  [unwired: 9 in]
  n134 = call "close_front_panel_in_exe.vi"("error_in"=w93, "vi_reference_in"=w92) -> ("error_out"=w91:errorcluster)  [unwired: 9 in]
  n135 = call <vilib>:"Clear Errors.vi"("error in (no error)"=w91) -> ()  [unwired: 5 in, 2 out]
